vi "功能测试.vi"(8 "error in (no error)":errorcluster caption="错误输入（无错误）") -> (0 "error out":errorcluster caption="错误输出")   [LabVIEW 2015]
doc: "该连续测量范例项目在队列消息处理器模板的基础上实现。\n\n事件处理循环负责按用户界面操作生成对应的消息。\n\n消息处理循环负责对事件处理循环或其他消息生成的消息进行处理。其中还包括用于采集和记录消息处理循环的子VI，以及用于更新图表的循环。"
uses:
  controls/UI Data.ctl
  Measure Type.ctl
  controls/ValueUI Data.ctl
  support/Message Queue/Enqueue Message (Single).vi
  Acquisition/Acquisition.lvlib
  Logging/Logging.lvlib
  support/User Event - Stop/User Event - Stop.lvlib
  support/Message Queue/Message Queue.lvlib
  Action/Action.lvlib
panel:
  out "XY Graph":cluster{"Y":dbl[], "Y":dbl[]}[](graph) caption="XY图"
  in  "设置":bool
  in  "清零":bool
  in  "读取":bool
  out "模拟通道5":dbl
  out "流量":dbl
  out "右推力":dbl
  out "左推力":dbl
  out "油压":dbl
  out "扭矩":dbl
  out "角度":dbl
  in  "计算":bool
  in  "Start":bool caption="开始"
  in  "Stop":bool caption="停止"
  out "Status":string caption="状态"
  in  "Exit":bool caption="退出"
  # "功能测试"
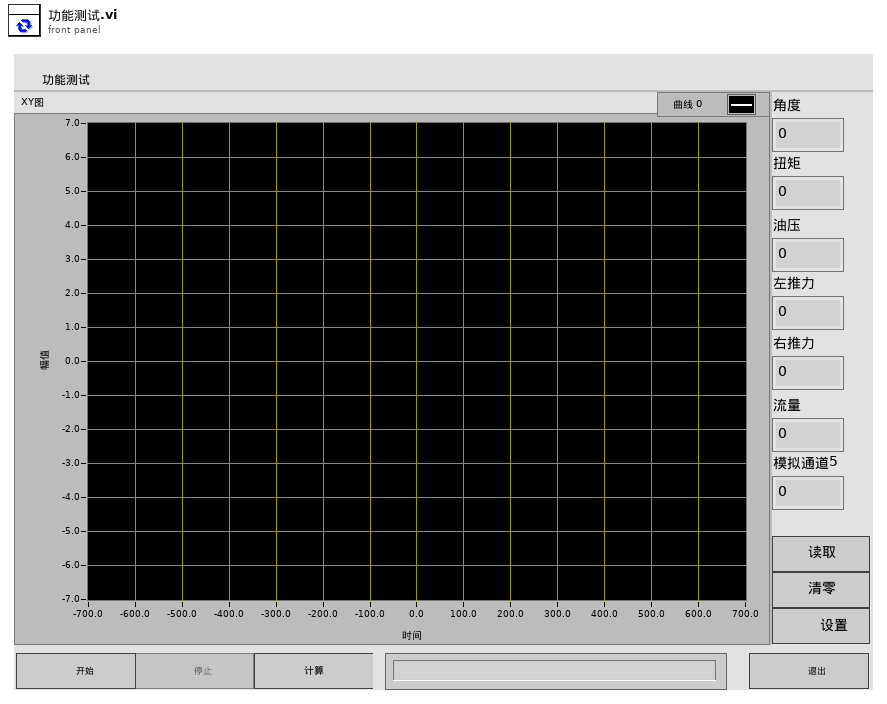
[diagram p1: front panel]
types:
  T1 = typedef "ValueUI Data.ctl" = cluster{"数据1引用":refnum<vi>, "数据2引用":refnum<vi>, "数据3引用":refnum<vi>, "传感器0引用":refnum<vi>, "传感器1引用":refnum<vi>, "传感器2引用":refnum<vi>, "传感器3引用":refnum<vi>, "传感器4引用":refnum<vi>, "传感器5引用":refnum<vi>, "传感器6引用":refnum<vi>}
  T2 = typedef "Measure Type.ctl" = enum16{"啮合", "退回", "功能", "力特性", "内泄漏", "自动调阀测试"}
  T3 = typedef "UI Data.ctl" = cluster{"Start Ref":refnum<vi>, "Stop Ref":refnum<vi>, "calculate Ref":refnum<vi>, "Status Ref":refnum<vi>, "Exit Ref":refnum<vi>, "read Ref":refnum<vi>, "clean Ref":refnum<vi>}
  T4 = typedef "Message Queue.lvlib/All Message Queues.ctl" = cluster{"UI":refnum<queue>, "Acquisition":refnum<queue>, "Logging":refnum<queue>, "plot logic":refnum<queue>, "Action Control":refnum<queue>}
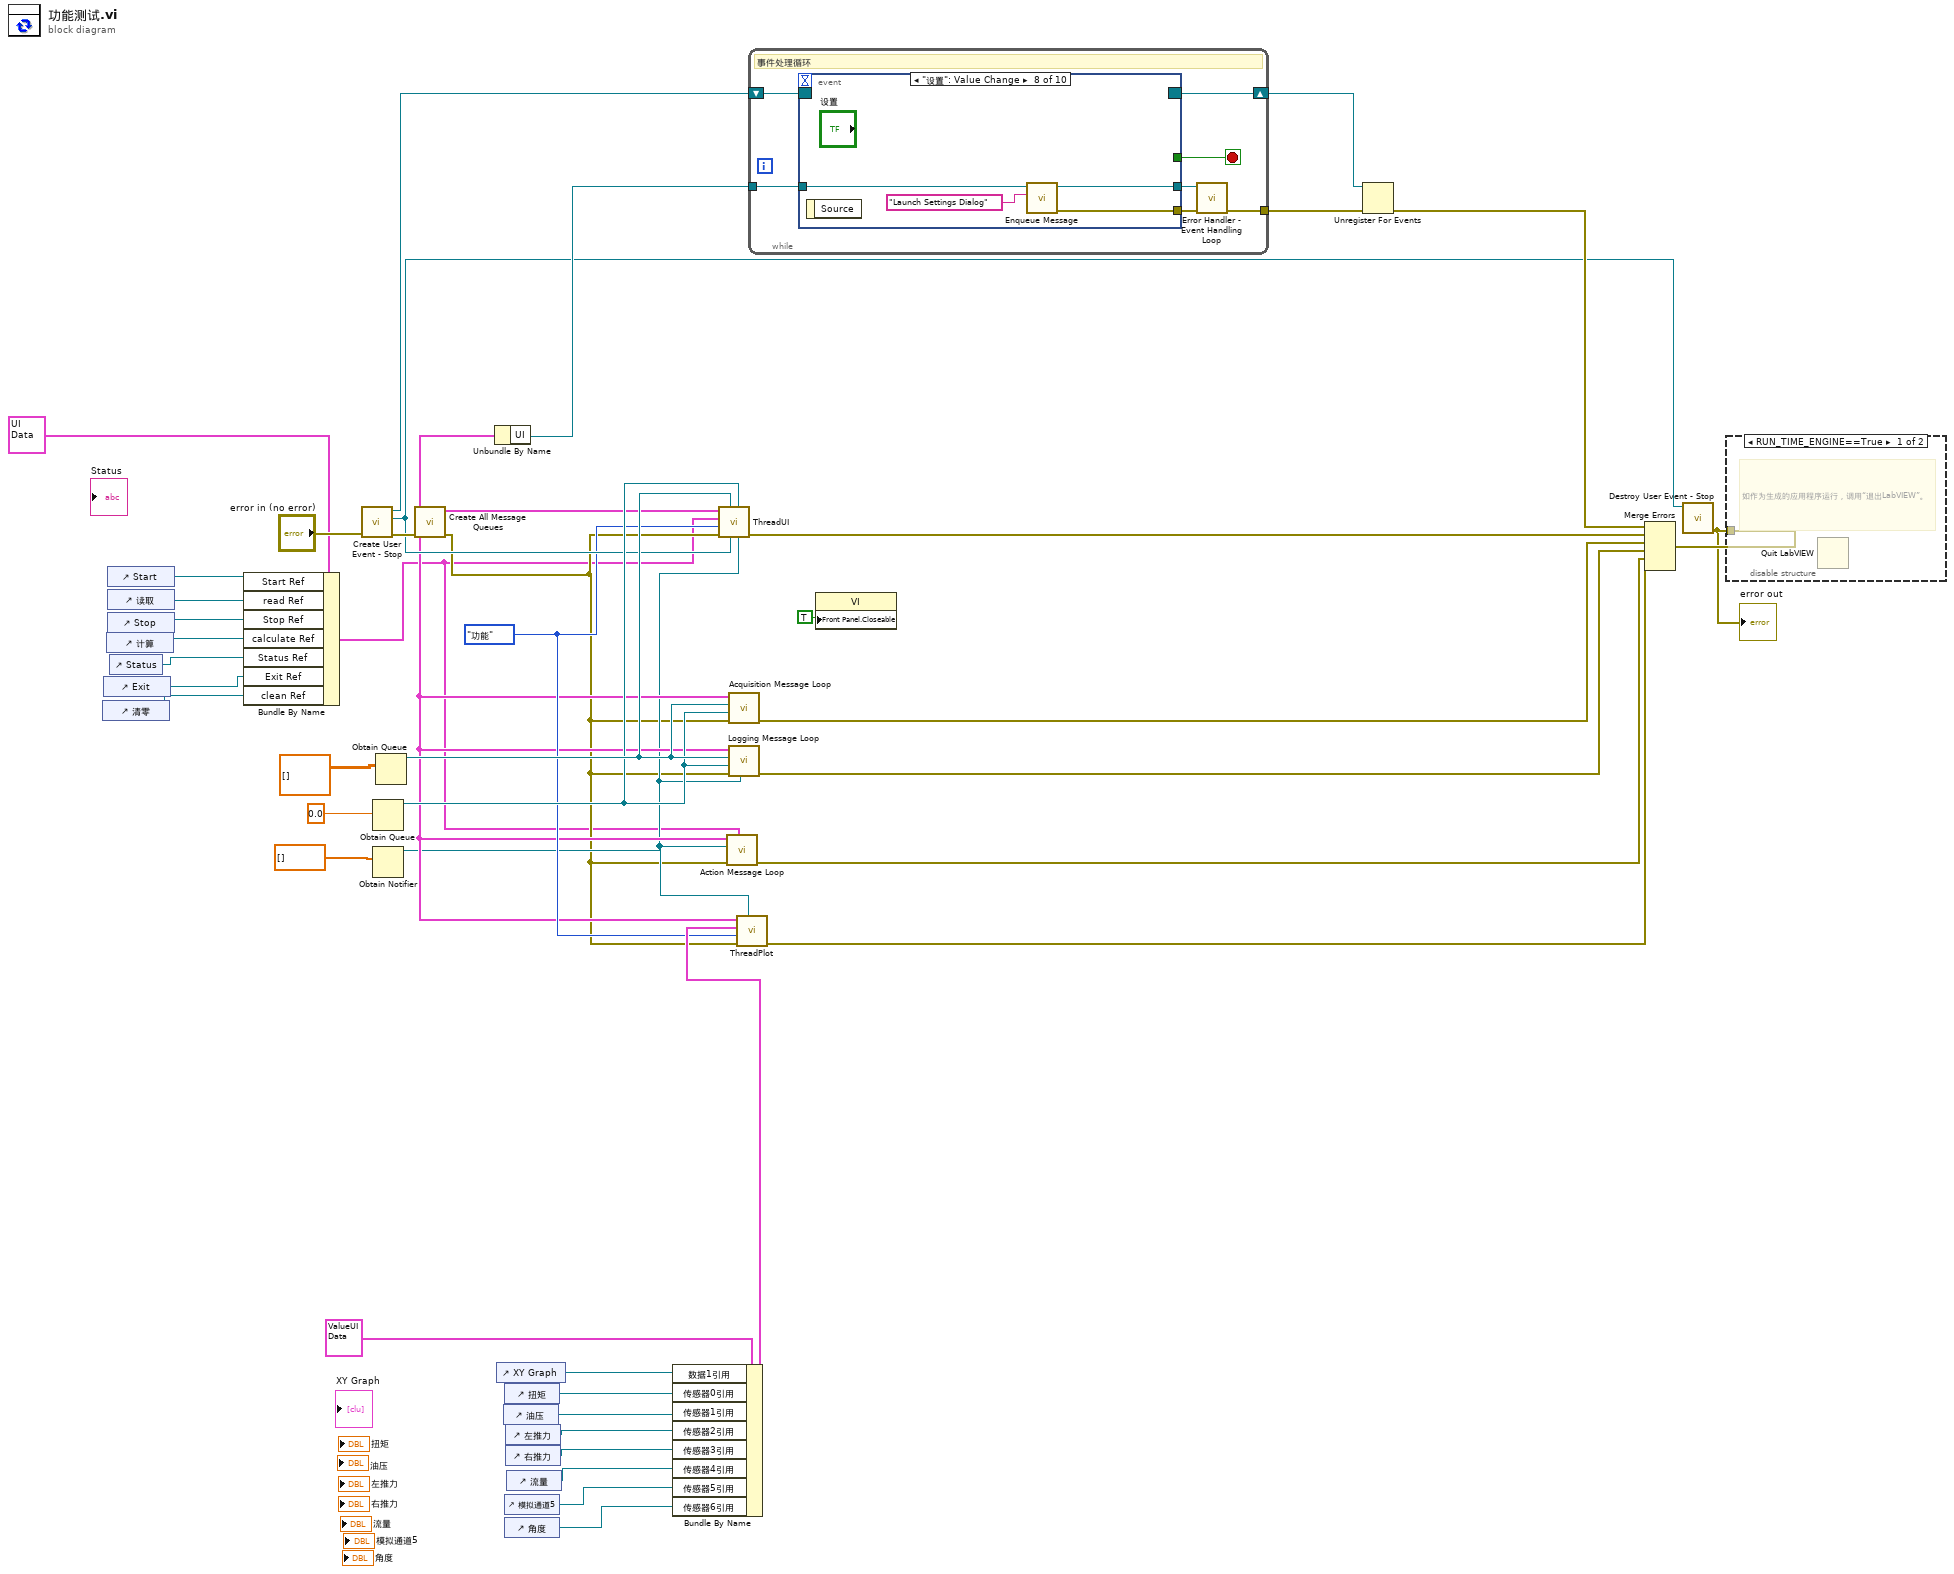
[diagram p0: block diagram]
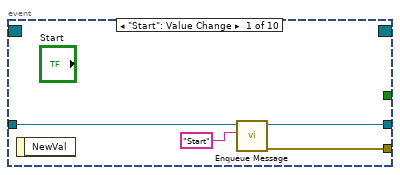
[diagram p3: hidden frame]
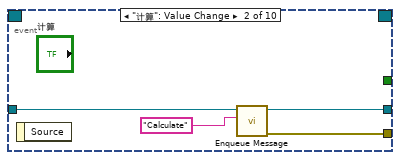
[diagram p4: hidden frame]
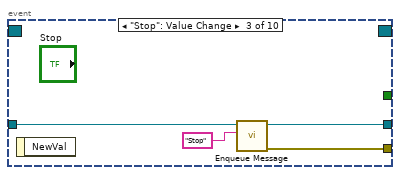
[diagram p5: hidden frame]
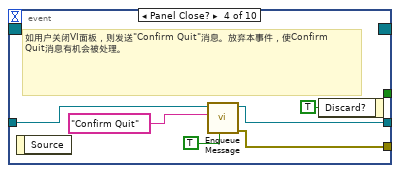
[diagram p6: hidden frame]
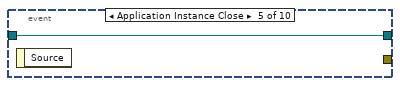
[diagram p7: hidden frame]
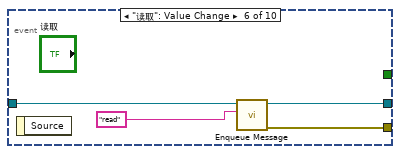
[diagram p8: hidden frame]
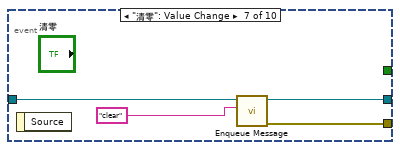
[diagram p9: hidden frame]
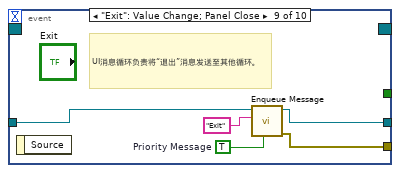
[diagram p10: hidden frame]
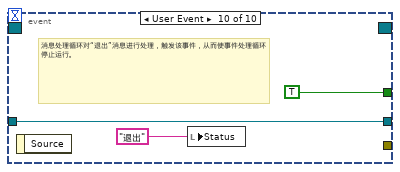
[diagram p11: hidden frame]
diagram:
  w8 = Measure_Type."功能" ("测试类型")
  n1 = control-ref of="清零"() -> (w25:refnum<vi>)
  n2 = control-ref of="Exit"() -> (w28:refnum<vi>)
  n3 = control-ref of="计算"() -> (w24:refnum<vi>)
  n4 = control-ref of="Start"() -> (w30:refnum<vi>)
  n5 = control-ref of="读取"() -> (w26:refnum<vi>)
  n6 = control-ref of="Stop"() -> (w27:refnum<vi>)
  n7 = control-ref of="Status"() -> (w6:refnum<vi>)
  n8 = Bundle By Name(cluster=T3 {"Start Ref"=refnum, "Stop Ref"=refnum, "calculate Ref"=refnum, "Status Ref"=refnum, "Exit Ref"=refnum, "read Ref"=refnum, "clean Ref"=refnum} ("Measurement UI Controls"), "Start Ref"=w30, "read Ref"=w26, "Stop Ref"=w27, "calculate Ref"=w24, "Status Ref"=w6, "Exit Ref"=w28, "clean Ref"=w25) -> (w2:T3)
  n9 = call "Create User Event - Stop.vi"("error in (no error)"="error in (no error)") -> ("error out"=w40:errorcluster, "User Event - Stop"=w20:refnum<user-event>, "Stop Event Registration Refnum"=w42:refnum<event-registration>)  [unwired: 8 in]
  n10 = Obtain Queue(element data type=0.0) -> (queue out=w22:refnum<queue>)  [unwired: 4 in, 2 out]
  n11 = Obtain Notifier(notification data type=dbl[] []) -> (notifier out=w4:refnum<notifier>)  [unwired: 3 in, 2 out]
  n12 = Obtain Queue(element data type=dbl[][] []) -> (queue out=w23:refnum<queue>)  [unwired: 4 in, 2 out]
  n13 = call "Create All Message Queues.vi"("error in (no error)"=w40) -> ("error out"=w3:errorcluster, "Message Queues out"=w5:T4)  [unwired: 9 in]
  n14 = Unbundle By Name(w5) -> ("UI"=w36:refnum<queue>)
  n15 = control-ref of="XY Graph"() -> (w17:refnum<vi>)
  n16 = control-ref of="油压"() -> (w15:refnum<vi>)
  n17 = control-ref of="扭矩"() -> (w16:refnum<vi>)
  n18 = control-ref of="模拟通道5"() -> (w11:refnum<vi>)
  n19 = control-ref of="角度"() -> (w10:refnum<vi>)
  n20 = control-ref of="左推力"() -> (w14:refnum<vi>)
  n21 = control-ref of="右推力"() -> (w13:refnum<vi>)
  n22 = control-ref of="流量"() -> (w12:refnum<vi>)
  n23 = Bundle By Name(cluster=T1 {"数据1引用"=refnum, "数据2引用"=refnum, "数据3引用"=refnum, "传感器0引用"=refnum, "传感器1引用"=refnum, "传感器2引用"=refnum, "传感器3引用"=refnum, "传感器4引用"=refnum, "传感器5引用"=refnum, "传感器6引用"=refnum} ("传感器显示UI控件"), "数据1引用"=w17, "传感器0引用"=w16, "传感器1引用"=w15, "传感器2引用"=w14, "传感器3引用"=w13, "传感器4引用"=w12, "传感器5引用"=w11, "传感器6引用"=w10) -> (w9:T1)
  n24 = call "ThreadUI.vi"("数据通知器"=w4, "Angle Data Queue"=w22, "User Event - Stop"=w20, "Analog Data Queue"=w23, "error in (no error)"=w3, "测试类型"=w8, "Measurement UI Controls"=w2, "Message Queues"=w5) -> ("error out"=w19:errorcluster)  [unwired: 3 in]
  n25 = call "Action Message Loop.vi"("Measurement UI Controls"=w2, "error in (no error)"=w3, "Data Notifier"=w4, "Message Queues"=w5) -> ("error out"=w1:errorcluster)  [unwired: 7 in]
  n26 = call "Acquisition Message Loop.vi"("error in (no error)"=w3, "Angle Data Queue"=w22, "Analog Data Queue"=w23, "Message Queues"=w5) -> ("error out"=w41:errorcluster)  [unwired: 7 in]
  n27 = call "Logging Message Loop.vi"("数据通知器"=w4, "error in (no error)"=w3, "Angle Data Queue"=w22, "Analog Data Queue"=w23, "Message Queues"=w5) -> ("error out"=w39:errorcluster)  [unwired: 6 in]
  n28 = call "ThreadPlot.vi"("数据通知器"=w4, "error in (no error)"=w3, "测试类型"=w8, "传感器显示UI控件"=w9, "Message Queues"=w5) -> ("error out"=w7:errorcluster)  [unwired: 6 in]
  n29 = while {
    tunnel: w36 -> [w50]
    tunnel: [w45] -> w44
    shift-right: [w49] -> w37
    shift-left: w42 -> [w51]
    stop <- w48 stop-if-true
    # "事件处理循环"
    n30 = event shown="[7] \"设置\": Value Change" {
      selector: w51 -> [_ _ _ _ _ _ _ _ _ _]
      dyn-events: [_ _ _ _ _ _ _ _ _ _] -> w49
      timeout: _ -> [_ _ _ _ _ _ _ _ _ _]
      tunnel: [_ _ _ _ _ _ _ _ _ TRUE ("Discard?")] -> w48
      tunnel: w50 -> [w53 w58 w62 w69 w70 w72 w76 w80 w84 w88]
      tunnel: [w55 w57 w61 w64 _ w74 w78 w82 w87 _] -> w46
      tunnel: [w52 w56 w60 w65 w70 w71 w75 w79 w83 w88] -> w47
      event "Start": Value Change {
        n31 = event-data() -> ()  [unwired: 1 in, 1 out]
        n32 = call-poly "Enqueue Message.vi"("Message"="Start", "Message Queue"=w53) -> ("error out"=w55:errorcluster, "dup Message Queue"=w52:refnum<queue>)  [unwired: 8 in]
      }
      event "计算": Value Change {
        n33 = event-data() -> ()  [unwired: 1 in, 1 out]
        n34 = call-poly "Enqueue Message.vi"("Message"="Calculate", "Message Queue"=w58) -> ("error out"=w57:errorcluster, "dup Message Queue"=w56:refnum<queue>)  [unwired: 8 in]
      }
      event "Stop": Value Change {
        n35 = event-data() -> ()  [unwired: 1 in, 1 out]
        n36 = call-poly "Enqueue Message.vi"("Message"="Stop", "Message Queue"=w62) -> ("error out"=w61:errorcluster, "dup Message Queue"=w60:refnum<queue>)  [unwired: 8 in]
      }
      event Panel Close? {
        # "如用户关闭VI面板，则发送\"Confirm Quit\"消息。放弃本事件，使Confirm Quit消息有机会被处理。"
        n37 = event-data() -> ()  [unwired: 1 in, 1 out]
        n38 = call-poly "Enqueue Message.vi"("Priority Message? (F)"=TRUE, "Message"="Confirm Quit", "Message Queue"=w69) -> ("error out"=w64:errorcluster, "dup Message Queue"=w65:refnum<queue>)  [unwired: 7 in]
        n39 = event-data("Discard?"=TRUE) -> ()  [unwired: 1 in, 1 out]
      }
      event Application Instance Close {
        n40 = event-data() -> ()  [unwired: 1 in, 1 out]
      }
      event "读取": Value Change {
        n41 = event-data() -> ()  [unwired: 1 in, 1 out]
        n42 = call-poly "Enqueue Message.vi"("Message"="read", "Message Queue"=w72) -> ("error out"=w74:errorcluster, "dup Message Queue"=w71:refnum<queue>)  [unwired: 8 in]
      }
      event "清零": Value Change {
        n43 = event-data() -> ()  [unwired: 1 in, 1 out]
        n44 = call-poly "Enqueue Message.vi"("Message"="clear", "Message Queue"=w76) -> ("error out"=w78:errorcluster, "dup Message Queue"=w75:refnum<queue>)  [unwired: 8 in]
      }
      event "设置": Value Change {
        n45 = event-data() -> ()  [unwired: 1 in, 1 out]
        n46 = call-poly "Enqueue Message.vi"("Message"="Launch Settings Dialog", "Message Queue"=w80) -> ("error out"=w82:errorcluster, "dup Message Queue"=w79:refnum<queue>)  [unwired: 8 in]
      }
      event "Exit": Value Change; Panel Close {
        w85 = TRUE  # Priority Message
        # "UI消息循环负责将“退出”消息发送至其他循环。"
        n47 = event-data() -> ()  [unwired: 1 in, 1 out]
        n48 = call-poly "Enqueue Message.vi"("Priority Message? (F)"=w85, "Message"="Exit", "Message Queue"=w84) -> ("error out"=w87:errorcluster, "dup Message Queue"=w83:refnum<queue>)  [unwired: 7 in]
      }
      event User Event {
        # "消息处理循环对“退出”消息进行处理，触发该事件，从而使事件处理循环停止运行。"
        n49 = event-data() -> ()  [unwired: 1 in, 1 out]
        n50 = local write "Status"("退出" ("Exit String")) -> ()
      }
    }
    n51 = call "Error Handler - Event Handling Loop.vi"("error in (no error)"=w46, "Message Queue"=w47) -> ("dup error in"=w45:errorcluster)  [unwired: 8 in, 1 out]
  }
  n52 = property class="VI"("Front Panel.Closeable"=TRUE ("Front Panel Window:Closeable")) -> ()  [unwired: 2 in, 2 out]
  n53 = Unregister For Events(event registration refnum=w37, error in=w44) -> (error out=w38:errorcluster)
  n54 = Merge Errors(w38, w19, w41, w39, w1, w7) -> (w43:errorcluster)
  n55 = call "Destroy User Event - Stop.vi"("error in (no error)"=w43, "User Event - Stop"=w20) -> ("error out"=w32:errorcluster)  [unwired: 9 in]
  "error out" <- w32
  n56 = disable-structure shown="RUN_TIME_ENGINE==True" {
    disable-tunnel: w32 -> [_ _]
    frame condition #0 {
      # "如作为生成的应用程序运行，调用“退出LabVIEW”。"
      n57 = Quit LabVIEW() -> ()  [unwired: 1 in]
    }
    frame condition #1 (active) {
    }
  }
